vi "标签.vi"(8 "错误输入（无错误）":errorcluster, 11 "引用":refnum<k24>) -> (0 "错误输出":errorcluster, 3 "引用输出":refnum<k24>)   [LabVIEW 2018]
uses:
  ScintillaNET.dll
  System.Drawing
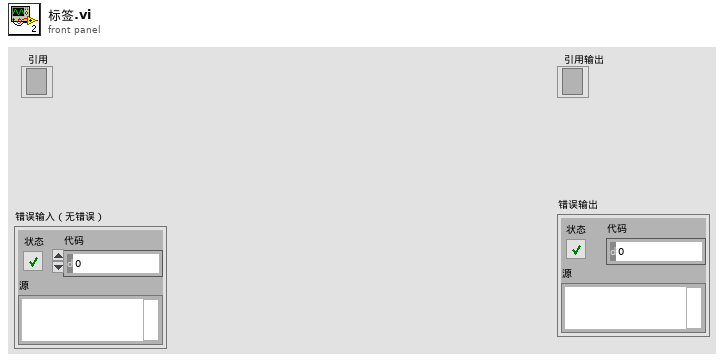
[diagram p1: front panel]
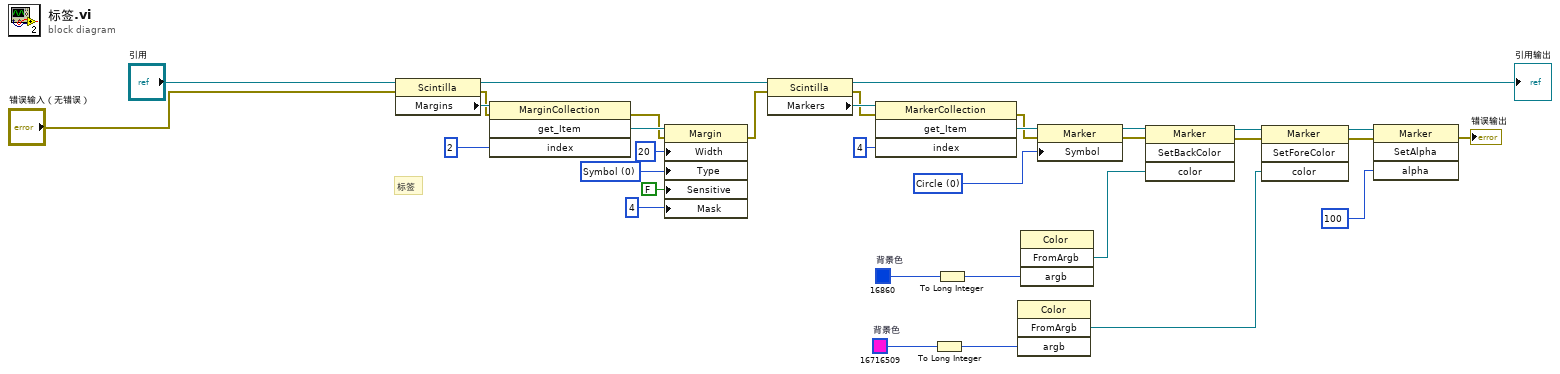
[diagram p0: block diagram]
diagram:
  w12 = u32 16716509  # 背景色
  w18 = u32 16860  # 背景色
  w22 = 0 items=["Circle"=0, "RoundRect"=1, "Arrow"=2, "SmallRect"=3, "ShortArrow"=4, "Empty"=5, "ArrowDown"=6, "Minus"=7, "Plus"=8, "VLine"=9, "LCorner"=10, "TCorner"=11, "BoxPlus"=12, "BoxPlusConnected"=13, "BoxMinus"=14, "BoxMinusConnected"=15, "LCornerCurve"=16, "TCornerCurve"=17, "CirclePlus"=18, "CirclePlusConnected"=19, "CircleMinus"=20, "CircleMinusConnected"=21, "Background"=22, "DotDotDot"=23, "Arrows"=24, "FullRect"=26, "LeftRect"=27, "Available"=28, "Underline"=29, "RgbaImage"=30, "Bookmark"=31] ("Symbol")
  w33 = 0 items=["Symbol", "Number", "BackColor", "ForeColor", "Text", "RightText", "Color"] ("Type")
  # "标签"
  n1 = property class="Scintilla"(reference="引用", error in="错误输入（无错误）") -> (reference out=w27:refnum<k24>, error out=w10:errorcluster, "Margins"=w28:refnum<k24>)
  n2 = invoke class="MarginCollection" method="get_Item"(reference=w28, error in=w10, "index"=2) -> (error out=w9:errorcluster, "get_Item"=w30:refnum<k24>)  [unwired: 1 in, 2 out]
  n3 = property class="Margin"(reference=w30, error in=w9, "Width"=20, "Type"=w33, "Sensitive"=FALSE, "Mask"=u32 4) -> (error out=w8:errorcluster)  [unwired: 1 out]
  n4 = property class="Scintilla"(reference=w27, error in=w8) -> (reference out=→"引用输出":refnum<k24>, error out=w7:errorcluster, "Markers"=w26:refnum<k24>)
  n5 = invoke class="MarkerCollection" method="get_Item"(reference=w26, error in=w7, "index"=4) -> (error out=w6:errorcluster, "get_Item"=w24:refnum<k24>)  [unwired: 1 in, 2 out]
  n6 = To Long Integer(number=w12) -> (32bit integer=w13:i32)
  n7 = To Long Integer(number=w18) -> (32bit integer=w17:i32)
  n8 = invoke class="Color" method="FromArgb"("argb"=w13) -> ("FromArgb"=w11:refnum<k24>)  [unwired: 3 in, 3 out]
  n9 = invoke class="Color" method="FromArgb"("argb"=w17) -> ("FromArgb"=w16:refnum<k24>)  [unwired: 3 in, 3 out]
  n10 = property class="Marker"(reference=w24, error in=w6, "Symbol"=w22) -> (reference out=w23:refnum<k24>, error out=w5:errorcluster)
  n11 = invoke class="Marker" method="SetBackColor"(reference=w23, error in=w5, "color"=w16) -> (reference out=w21:refnum<k24>, error out=w4:errorcluster)  [unwired: 1 in, 2 out]
  n12 = invoke class="Marker" method="SetForeColor"(reference=w21, error in=w4, "color"=w11) -> (reference out=w20:refnum<k24>, error out=w3:errorcluster)  [unwired: 1 in, 2 out]
  n13 = invoke class="Marker" method="SetAlpha"(reference=w20, error in=w3, "alpha"=100) -> (error out=→"错误输出":errorcluster)  [unwired: 1 in, 3 out]
